vi "VI_find_salt.vi"(6 "LVSR block":string, 8 "error in (no error)":errorcluster, 9 "Hash1 (MD5)":string, 10 "Hash1 raw (no salt)":string, 11 "VCTP block":string) -> (0 "error out":errorcluster, 3 "Salt":string)   [LabVIEW 2023]
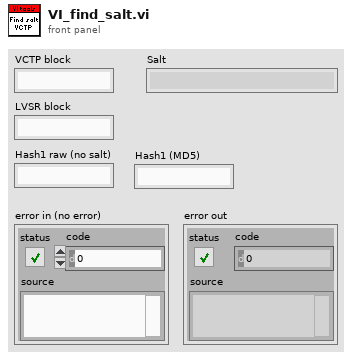
[diagram p1: front panel]
types:
  T1 = enum16{"big-endian, network order", "native, host order", "little-endian"}
  T2 = cluster{"Numbers":i32, "Strings":i32, "Paths":i32}
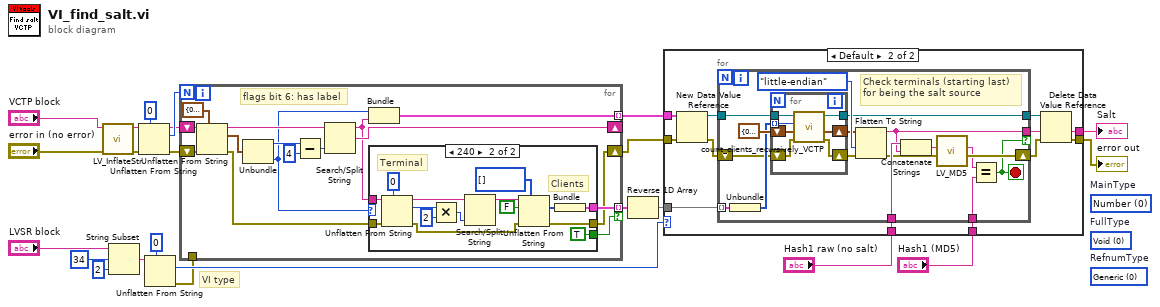
[diagram p0: block diagram]
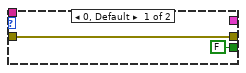
[diagram p2: hidden frame]
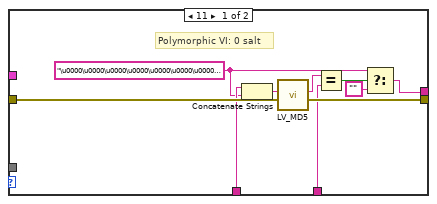
[diagram p3: hidden frame]
diagram:
  (unwired) u8 0 items=["Generic"=0, "DataLog"=1, "ByteStream"=2, "Device"=3, "Occurrence"=4, "TCPNetConn"=5, "AutoRef"=7, "LVObjCtl"=8, "Menu"=9, "Imaq"=11, "DataSocket"=13, "VisaRef"=14, "IVIRef"=15, "UDPNetConn"=16, "NotifierRef"=17, "Queue"=18, "IrdaNetConn"=19, "UsrDefined"=20, "UsrDefndTag"=21, "EventReg"=23, "DotNet"=24, "UserEvent"=25, "Callback"=27, "UsrDefTagFlt"=29, "UDClassInst"=30, "BluetoothCon"=31, "DataValueRef"=32, "FIFORef"=33, "TDMSFile"=34]  # RefnumType
  (unwired) u8 0 items=["Void"=0, "NumberI8"=1, "NumberI16"=2, "NumberI32"=3, "NumberI64"=4, "NumberU8"=5, "NumberU16"=6, "NumberU32"=7, "NumberU64"=8, "NumberSGL"=9, "NumberDBL"=10, "NumberEXT"=11, "NumberCSG"=12, "NumberCDB"=13, "NumberCXT"=14, "UnitI8"=17, "UnitI16"=18, "UnitI32"=19, "UnitI64"=20, "UnitU8"=21, "UnitU16"=22, "UnitU32"=23, "UnitU64"=24, "UnitSGL"=25, "UnitDBL"=26, "UnitEXT"=27, "UnitCSG"=28, "UnitCDB"=29, "UnitCXT"=30, "BoolU16"=32, "Bool"=33, "String"=48, "String2"=49, "Path"=50, "Picture"=51, "CString"=52, "PascalString"=53, "Tag"=55, "SubString"=63, "Array"=64, "ArrayDataPtr"=65, "SubArray"=79, "Cluster"=80, "LVVariant"=83, "MeasureData"=84, "ComplexFixedPt"=94, "FixedPoint"=95, "Block"=96, "TypeBlock"=97, "VoidBlock"=98, "AlignedBlock"=99, "RepeatedBlock"=100, "AlignmntMarker"=101, "Refnum"=112, "Set"=115, "Map"=116, "PointerNumber"=128, "PointerNumberI8"=129, "PointerNumberI16"=130, "PointerNumberI32"=131, "PointerNumberI64"=132, "PointerNumberU8"=133, "PointerNumberU16"=134, "PointerNumberU32"=135, "PointerNumberU64"=136, "PointerNumberSGL"=137, "PointerNumberDBL"=138, "PointerNumberEXT"=139, "PointerNumberCSG"=140, "PointerNumberCDB"=141, "PointerNumberCXT"=142, "ArrayInterfc"=160, "InterfcToData"=161, "Terminal"=240, "TypeDef"=241, "PolyVI"=242]  # FullType
  (unwired) u8 0 items=["Number"=0, "Unit"=1, "Bool"=2, "Blob"=3, "Array"=4, "Cluster"=5, "Block"=6, "Refnum"=7, "NumberPointer"=8, "Terminal"=15]  # MainType
  # "VI type"
  n1 = call "LV_InflateStr.vi"("error in (no error)"="error in (no error)", "Deflated string with size header"="VCTP block") -> ("error out"=w17:errorcluster, "Inflated string"=w20:string)  [unwired: 8 in]
  n2 = String Subset(string="LVSR block", offset (0)=34, length (rest)=2 ("length (rest)")) -> (substring=w5:string)
  n3 = Unflatten From String(type=0, binary string=w20, error in (no error)=w17) -> (rest of the binary string=w21:string, value=w22:i32, error out=w16:errorcluster)  [unwired: 2 in]
  n4 = Unflatten From String(type=u16 0 ("viType"), binary string=w5) -> (value=w2:u16, error out=w1:errorcluster)  [unwired: 3 in, 1 out]
  n5 = for {
    N: w22 -> [_]
    shift-right: [w34] -> _
    shift-left: w21 -> [w39]
    tunnel: [w32] -> w15 mode=indexing
    tunnel: [w28] -> w14 mode=indexing if=w24
    shift-right: [w26] -> w12
    shift-left: w16 -> [w29]
    tunnel: w1 -> [_]
    # "flags bit 6: has label"
    n6 = Unflatten From String(type=cluster{"length":i16, "flags":u8, "type":u8} {"length"=0, "flags"=0, "type"=0}, binary string=w39, error in (no error)=w29) -> (rest of the binary string=w36:string, value=w37:cluster{"length":i16, "flags":u8, "type":u8}, error out=w27:errorcluster)  [unwired: 2 in]
    n7 = Unbundle(w37) -> ("length"=w33:i16, "type"=w25:u8)  [unwired: 1 out]
    n8 = Subtract(x=w33, y=i16 4) -> (x-y=w35:i16)
    n9 = Search/Split String(string=w36, offset (0)=w35) -> (substring before match=w30:string, match + rest of string=w34:string)  [unwired: 1 in, 1 out]
    n10 = Bundle("type"=w25, w30) -> (w32:cluster{"type":u8, string})  [unwired: 1 in]
    n11 = case shown="240" w25 {
      tunnel: w30 -> [_ w49]
      tunnel: [_ w47] -> w28
      tunnel: w27 -> [w41 w46]
      tunnel: [w41 w44] -> w26
      tunnel: [FALSE TRUE] -> w24
      frame 0, Default {
      }
      frame 240 {
        # "Terminal"
        # "Clients"
        n12 = Unflatten From String(type=i16 0, binary string=w49, error in (no error)=w46) -> (rest of the binary string=w53:string, value=w55:i16, error out=w45:errorcluster)  [unwired: 2 in]
        n13 = Multiply(x=w55, y=i16 2) -> (x*y=w52:i16)
        n14 = Search/Split String(string=w53, offset (0)=w52) -> (substring before match=w50:string)  [unwired: 1 in, 2 out]
        n15 = Unflatten From String(type=i16[] [] ("index"), binary string=w50, data includes array or string size? (T)=FALSE, error in (no error)=w45) -> (value=w48:i16[], error out=w44:errorcluster)  [unwired: 1 in, 1 out]
        n16 = Bundle("index"=w48) -> (w47:cluster{"index":i16[]})  [unwired: 1 in]
      }
    }
  }
  n17 = Reverse 1D Array(array=w14) -> (reversed array=w13:cluster{"index":i16[]}[])
  n18 = case shown="Default" w2 {
    tunnel: w13 -> [_ w77]
    tunnel: w15 -> [_ w76]
    tunnel: w12 -> [w64 w73]
    tunnel: [w57 w70] -> w11
    tunnel: [w62 w69] -> w10
    tunnel: "Hash1 (MD5)" -> [w61 w68]
    tunnel: "Hash1 raw (no salt)" -> [w63 w67]
    frame 11 {
      w59 = "\u0000\u0000\u0000\u0000\u0000\u0000\u0000\u0000\u0000\u0000\u0000\u0000" ("Salt")
      # "Polymorphic VI: 0 salt"
      n19 = Concatenate Strings(w63, w59) -> (w66:string)
      n20 = call "LV_MD5.vi"("error in (no error)"=w64, "Input string"=w66) -> ("error out"=w62:errorcluster, "MD5 digest (16-bytes)"=w65:string)  [unwired: 8 in]
      n21 = Equal?(x=w65, y=w61) -> (x = y?=w60:bool)
      n22 = Select(t=w59, s=w60, f="") -> (s? t:f=w57:string)
    }
    frame Default {
      n23 = New Data Value Reference(data value=w76, error in=w73) -> (data value reference=w75:refnum<data-value>, error out=w74:errorcluster)
      n24 = for {
        tunnel: w77 -> [w91] mode=indexing
        tunnel: w75 -> [w89]
        shift-right: [w82] -> w71
        shift-left: w74 -> [w88]
        tunnel: [w86] -> w72
        tunnel: w67 -> [w85]
        tunnel: w68 -> [w80]
        tunnel: [w79] -> w70 if=w78
        stop <- w78 stop-if-true
        # "Check terminals (starting last)\nfor being the salt source"
        n25 = Unbundle(w91) -> ("index"=w90:i16[])
        n26 = for {
          tunnel: w90 -> [w100] mode=indexing
          shift-right: [w101] -> w92
          shift-left: T2 {"Numbers"=0, "Strings"=0, "Paths"=0} ("Control counts out") -> [w99]
          tunnel: [w98] -> w86
          shift-right: [w97] -> w87
          shift-left: w88 -> [w96]
          tunnel: w89 -> [w95]
          n27 = call "count_clients_recursively_VCTP.vi"("error in (no error)"=w96, "Control counts in (0)"=w99, "Type descriptor index"=w100, "VCTP type descriptor list"=w95) -> ("error out"=w97:errorcluster, "Control counts out"=w101:T2, "Type descriptor list dup"=w98:refnum<data-value>)  [unwired: 5 in]
        }
        n28 = Flatten To String(anything=w92, byte order (0:big-endian, network order)=T1."little-endian", error in (no error)=w87) -> (data string=w79:string, error out=w83:errorcluster)  [unwired: 1 in, 1 out]
        n29 = Concatenate Strings(w85, w79) -> (w84:string)
        n30 = call "LV_MD5.vi"("error in (no error)"=w83, "Input string"=w84) -> ("error out"=w82:errorcluster, "MD5 digest (16-bytes)"=w81:string)  [unwired: 8 in]
        n31 = Equal?(x=w81, y=w80) -> (x = y?=w78:bool)
      }
      n32 = Delete Data Value Reference(data value reference=w72, error in=w71) -> (error out=w69:errorcluster)  [unwired: 1 out]
    }
  }
  "Salt" <- w11
  "error out" <- w10
